vi "ManipSetPreloadBalls.vi"(11 "Parameter String":string) -> (1 "Error Out":errorcluster, 3 "Increment":bool)   [LabVIEW 2020]
uses:
  SafeParser_Integer.vi
  sensordata.vi
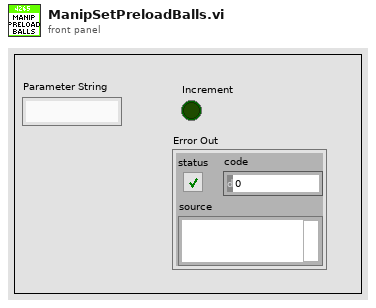
[diagram p1: front panel]
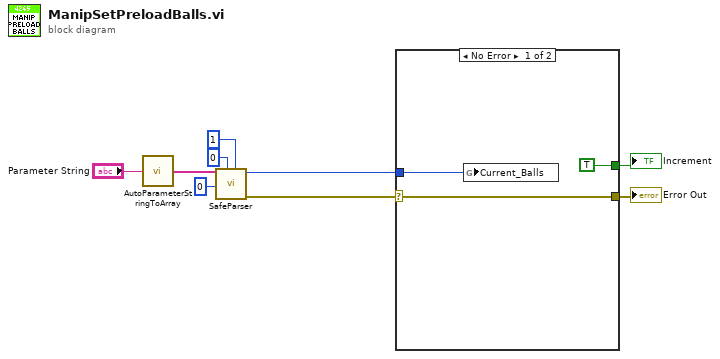
[diagram p0: block diagram]
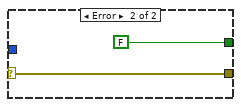
[diagram p2: hidden frame]
diagram:
  n1 = call "AutoParameterStringToArray.vi"("Parameter String"="Parameter String") -> ("Parsed Parameters"=w4:string[])
  n2 = call-poly "SafeParser.vi"("Maximum"=1, "Minimum"=0, "Array Index"=0 ("Parameter Index"), "String Array"=w4) -> ("Error Out"=w1:errorcluster, "Typecast  Value"=w6:i32)  [unwired: 6 in]
  n3 = case shown="No Error" w1 {
    selector: w1 -> [w12 w14]
    tunnel: [TRUE FALSE] -> w9
    tunnel: [w12 w14] -> w8
    tunnel: w6 -> [w10 _]
    frame No Error {
      n4 = global write "sensordata.vi" "Current_Balls"(w10) -> ()
    }
    frame Error {
    }
  }
  "Increment" <- w9
  "Error Out" <- w8
